vi "GenerateDMDcalibMASKS.vi"() -> ()   [LabVIEW 2017]
panel:
  in  "path to BMP file":path=path "\\\\LEO1272\\Caplins/Calibrations/MASKS"
  in  "radius":i16=5
  in  "N_Y":i32=6
  in  "N_X":i32=6
  in  "y0":i32=250
  in  "x0":i32=300
  in  "dY":i32=64
  in  "dX":i32=64
  out "empty picture":picture
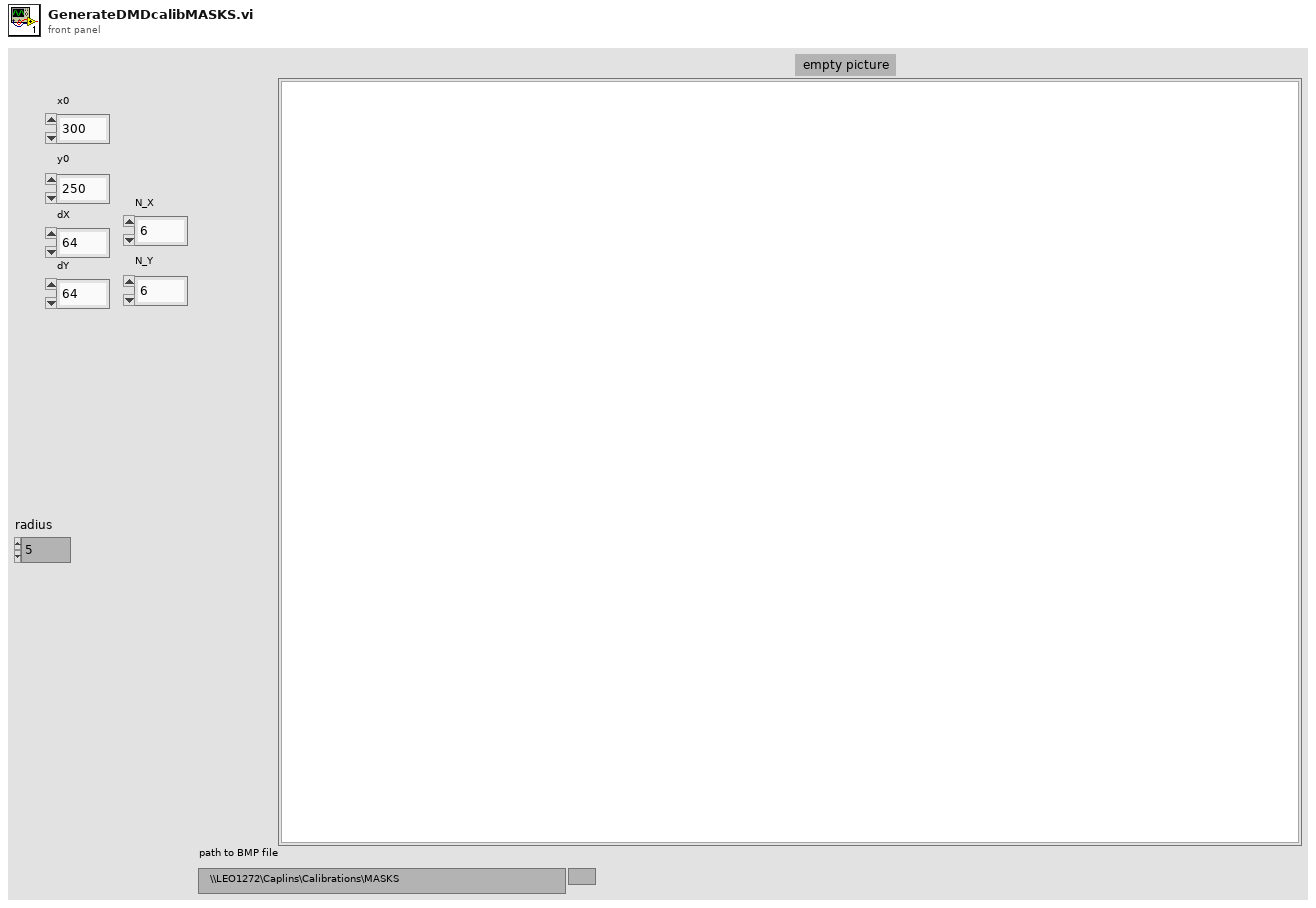
[diagram p1: front panel]
types:
  T1 = cluster{"y0 2":i32, "y0 2":i32, "y0 2":i32, "y0 2":i32}
  T2 = typedef "imagedata.ctl" = cluster{"image type":i32, "image depth":i32, "image":u8[], "mask":u8[], "colors":u32[], "Rectangle":cluster{"left":i16, "top":i16, "right":i16, "bottom":i16}}
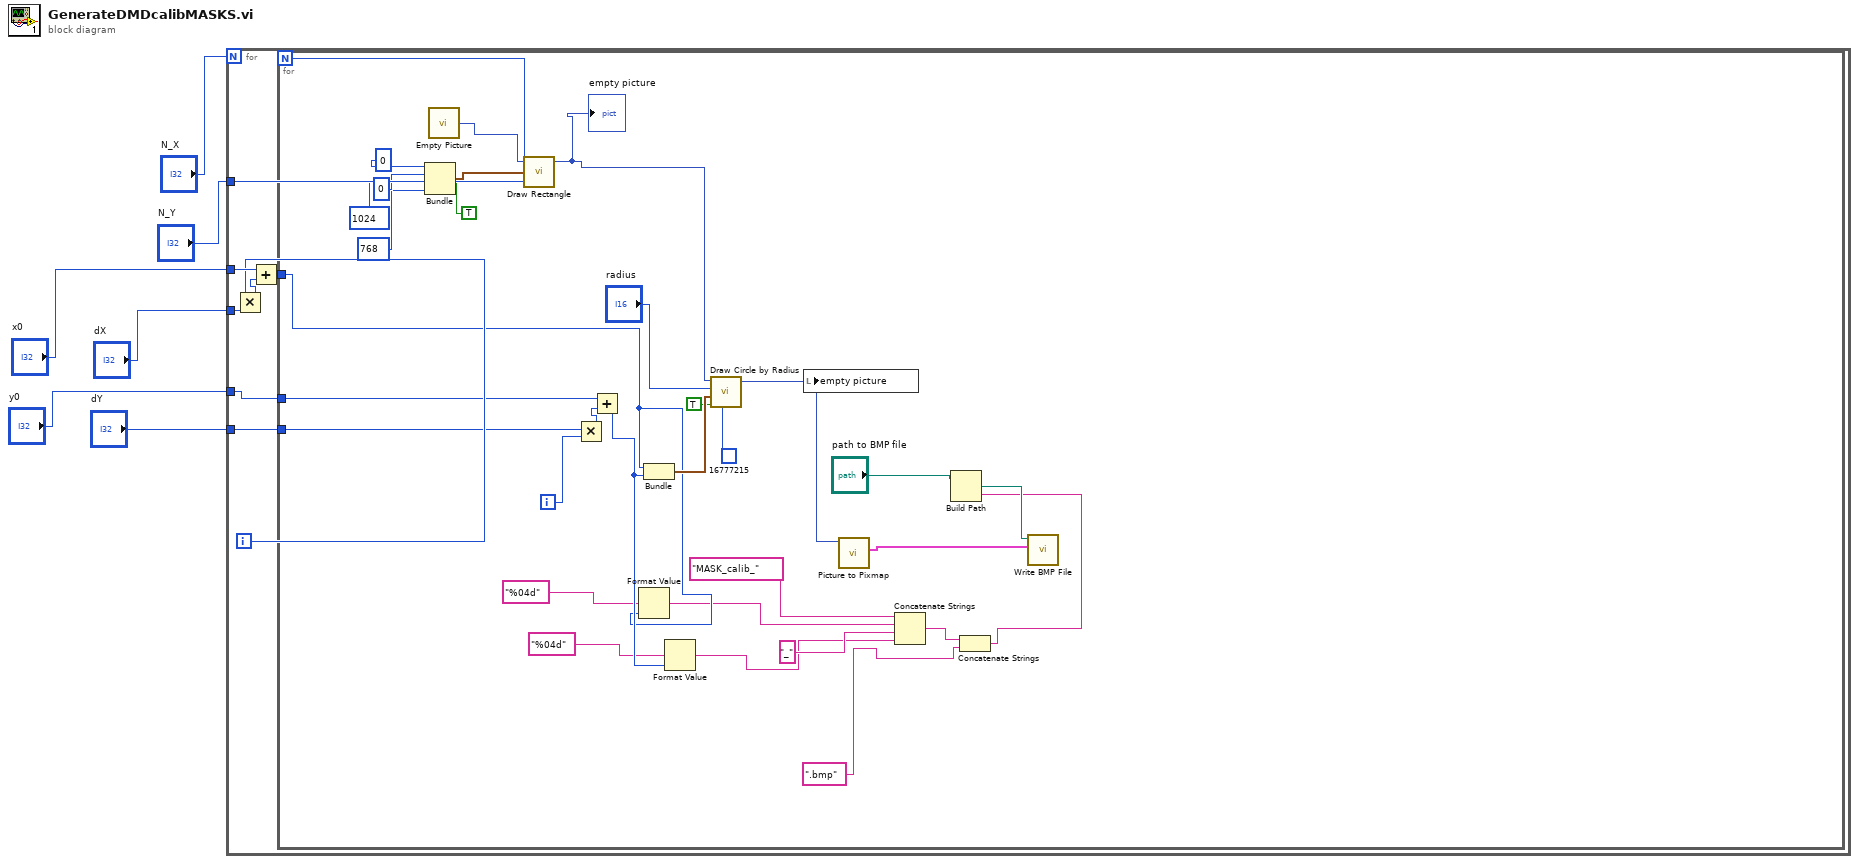
[diagram p0: block diagram]
diagram:
  n1 = for {
    N: "N_X" -> [_]
    tunnel: "x0" -> [w13]
    tunnel: "dX" -> [w12]
    tunnel: "y0" -> [w8]
    tunnel: "dY" -> [w7]
    tunnel: "N_Y" -> [w14]
    i -> [w11]
    n2 = Multiply(x=w11, y=w12) -> (x*y=w10:i32)
    n3 = Add(x=w13, y=w10) -> (x+y=w9:i32)
    n4 = for {
      N: w14 -> [_]
      tunnel: w9 -> [w17]
      tunnel: w8 -> [w45]
      tunnel: w7 -> [w44]
      i -> [w43]
      n5 = Bundle("y0 2"=0, "y0 2"=0, "y0 2"=1024, "y0 2"=768) -> (w36:T1)  [unwired: 1 in]
      n6 = call "Empty Picture"() -> ("empty picture"=w37:picture)
      n7 = call <vilib>:"Draw Rectangle.vi"("picture"=w37, "rect"=w36, "fill?(F)"=TRUE) -> ("new picture"=w30:picture)  [unwired: 6 in]
      "empty picture" <- w30
      n8 = Multiply(x=w44, y=w43) -> (x*y=w42:i32)
      n9 = Add(x=w45, y=w42) -> (x+y=w20:i32)
      n10 = Format Value(format string="%04d", value (0)=w17) -> (output string=w16:string)  [unwired: 1 in]
      n11 = Bundle(w17, w20) -> (w40:cluster{i32, i32})  [unwired: 1 in]
      n12 = Format Value(format string="%04d", value (0)=w20) -> (output string=w15:string)  [unwired: 1 in]
      n13 = call <vilib>:"Draw Circle by Radius.vi"("color(black)"=u32 16777215, "fill?(F)"=TRUE, "pixel center"=w40, "radius"="radius", "picture"=w30) -> ("new picture"=w28:picture)  [unwired: 6 in]
      n14 = local write "empty picture"(w28) -> ()
      n15 = call <vilib>:"Picture to Pixmap.vi"("picture"=w28) -> ("image data"=w29:T2)  [unwired: 9 in, 1 out]
      n16 = Concatenate Strings("MASK_calib_" ("string"), w16, "_" ("string"), w15) -> (w22:string)
      n17 = Concatenate Strings(w22, ".bmp" ("string")) -> (w21:string)
      n18 = Build Path(base path="path to BMP file", name or relative path=w21) -> (appended path=w24:path)
      n19 = call <vilib>:"Write BMP File.vi"("image data"=w29, "path to BMP file"=w24) -> ()  [unwired: 8 in, 2 out]
    }
  }
